vi "Q14070-Z050在线跑合.vi"() -> ()   [LabVIEW 2013]
panel:
  in  "确定按钮 3":bool
  in  "确定按钮 2":bool
  in  "密码":string
  in  "确定按钮":bool
  out "不合格":bool
  out "error out 4":errorcluster
  out "error out":errorcluster
  out "Data":string[][](array[string])
  out "型号数量":i32=10
  out "通道0":dbl
  out "I复位按钮":bool
  out "I急停按钮":bool
  out "报警信息":string
  out "电机当前位置":dbl=10000.0 format="%#.2f"
  out "拉压力（N）":dbl format="%#.1f"
  out "通讯状态":bool
  in  "停止":bool
  out "自动操作状态":string
  out "工步号":dbl
  in  "联线按钮":bool
  in  "选项卡控件 2":enum32{"自动工步", "手动气缸", "传感器校验", "参数查询"}(tab)
  out "跑和设定百分比":dbl=3.0 format="%#_2f"
  out "跑和百分比":dbl=1.0 format="%.2f"
  out "跑合已完成次数":dbl
  out "跑合速度(mm/s)":dbl=3.0 format="%#_2f"
  out "跑合设定次数":dbl=10.0
  out "左极限位置(mm)":dbl=-40.0
  out "右极限位置(mm)":dbl=60.0
  out "齿条中心位置（mm)":dbl=14.0
  out "齿条行程(mm)":dbl=14.0
  out "顶升气缸上位 2":bool
  out "顶升气缸下位 2":bool
  out "齿条夹紧 2":bool
  out "齿条松开 2":bool
  out "下工位在位  2":bool
  out "本工位在位 2":bool
  out "上工位在位  2":bool
  out "换向拉压力(N)":dbl format="%#.3f"
  out "本序合格":bool
  out "上序不合格":bool
  out "上序合格":bool
  out "本序已做":bool
  out "I齿条松开":bool
  out "I齿条夹紧":bool
  out "I顶升气缸下位":bool
  out "I顶升气缸上位":bool
  out "下工位在位":bool
  out "本工位在位":bool
  out "上工位在位":bool
  in  "M上阻挡器放行":bool
  in  "M本阻挡器放行":bool
  in  "M顶升气缸上升":bool
  in  "M顶升气缸下降":bool
  in  "M齿条气缸夹紧":bool
  in  "M齿条气缸松开":bool
  in  "电机前进":bool
  in  "电机后退":bool
  in  "电机回零":bool
  in  "拉压力1传感器零点偏移":dbl format="%#.2f"
  in  "拉压力1传感器比例偏移":dbl=1.0 format="%#.2f"
  in  "传感器参数保存":bool
  in  "参数查询":bool
  in  "参数列表":string[][](table)
  in  "参数修改":bool
  out "员工ID":string
  out "员工姓名":string
  in  "型号选择":u16(ring)=1 items=["J706", "J709", "J728"]
  in  "参数加载":bool
  out "产品ID":string
  out "报警 工步号":dbl
  out "完成":bool
  out "error out 3":errorcluster
  out "芯片ID":string
  out "error out 2":errorcluster
  out "ADODB._Connection Out":refnum<k7>
  out "跑合曲线":cluster{dbl[], dbl[]}(graph)
  out "FGCS":string
  out "RFID读取完成":bool
  out "RFID读取触发":bool
  out "05RFID":string
  out "KSJJ":string
  out "ReturnValue 3":u32
  out "ReturnValue":u32
  out "轴1AxisHandle OUT":u32
  out "DeviceHandle":u32
  # "芜湖机械转向器装配线"
  # "在线跑合"
  # "湖北唯思凌科装备制造有限公司 设计开发 (C)2015"
  # "Q14070机械转向器装配线"
  # "传感器校验区"
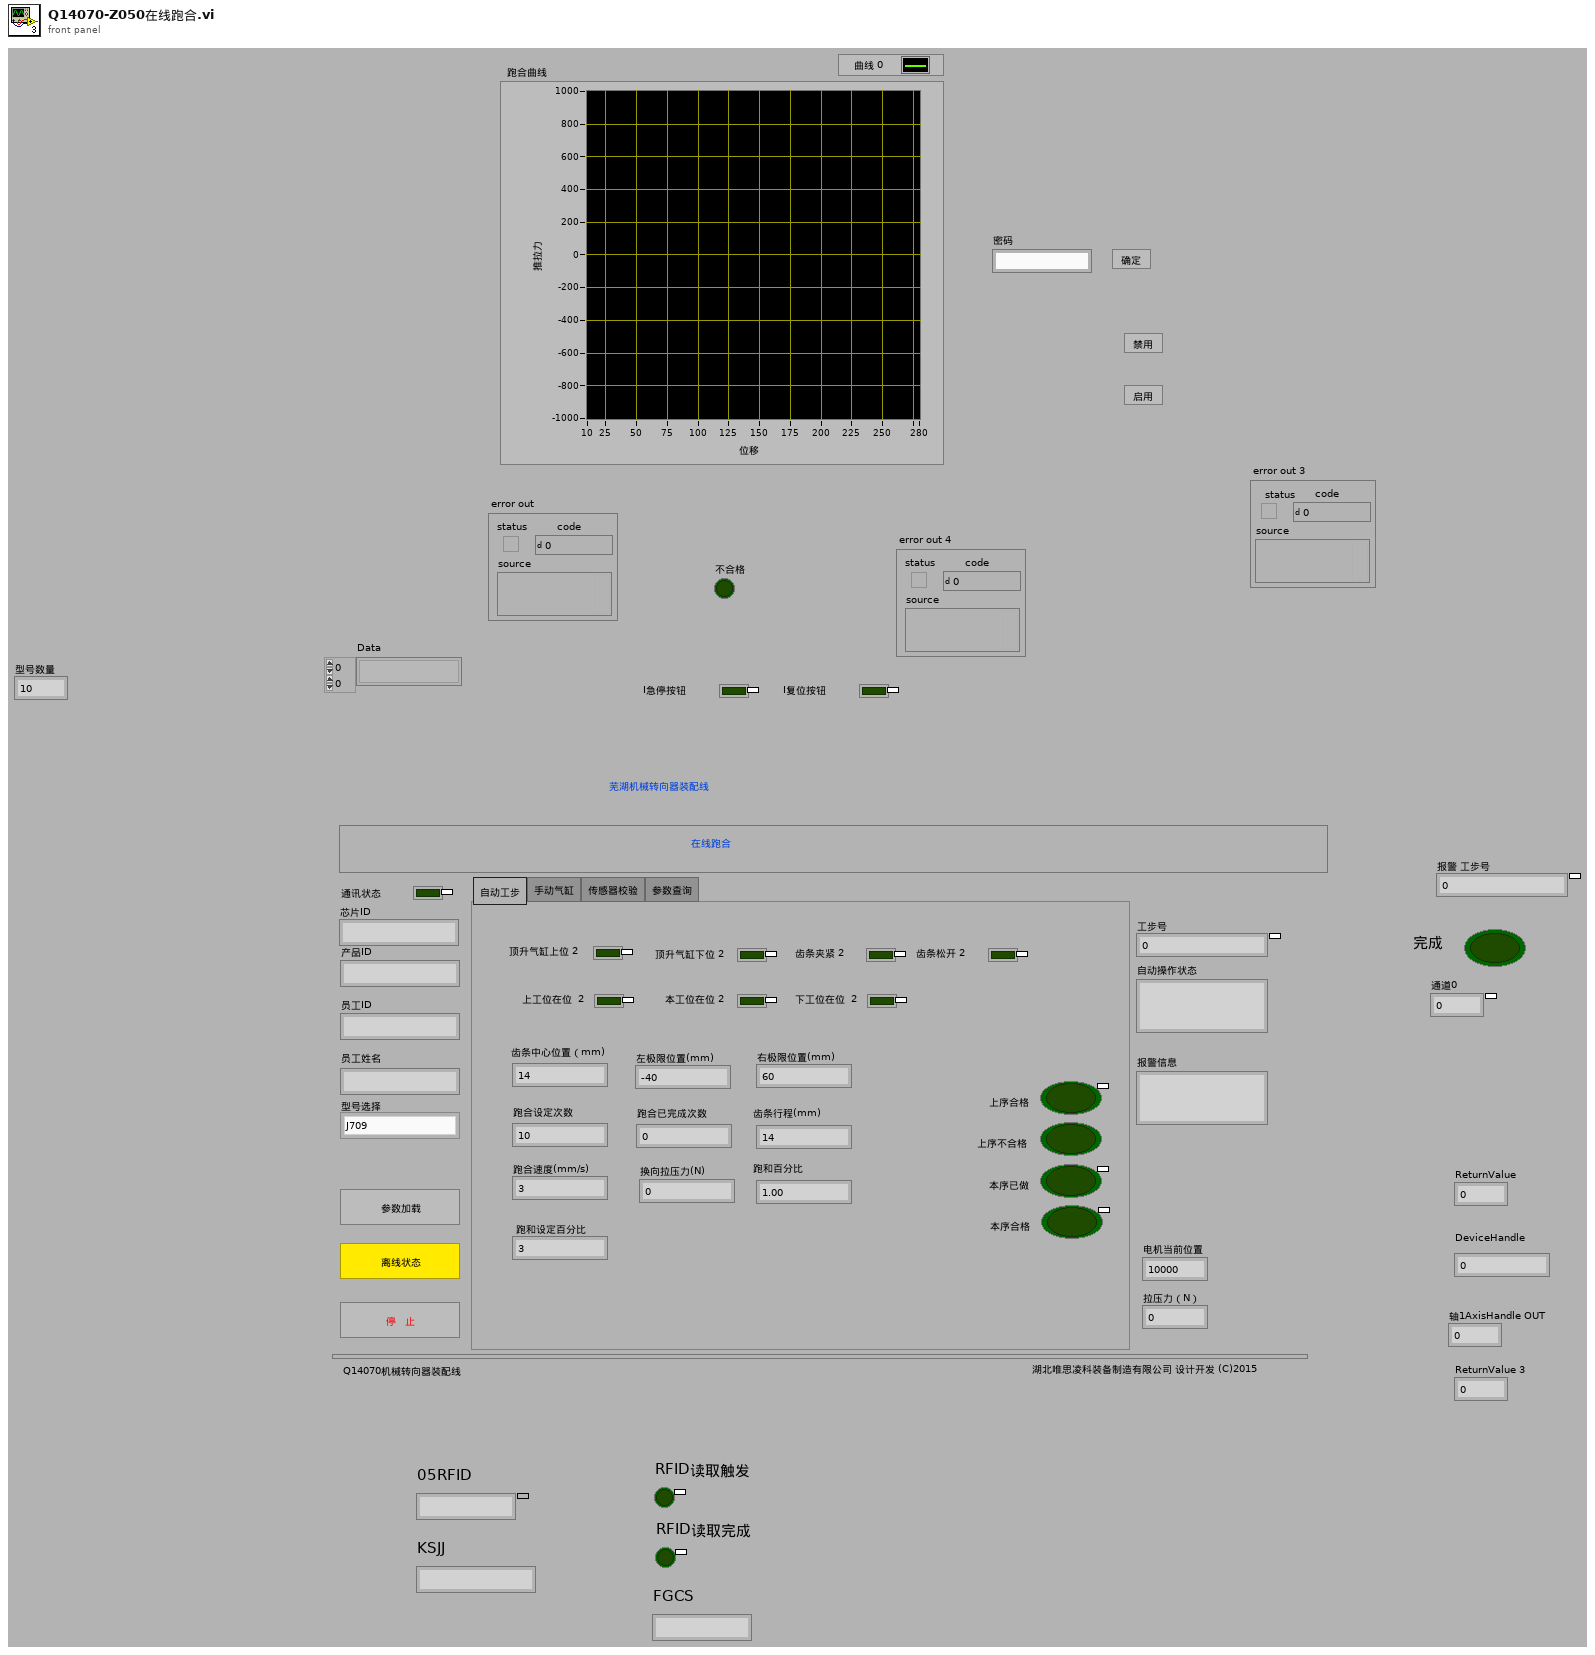
[diagram p1: front panel]
types:
  T1 = enum8{"Enabled", "Disabled", "Disabled and Grayed Out"}
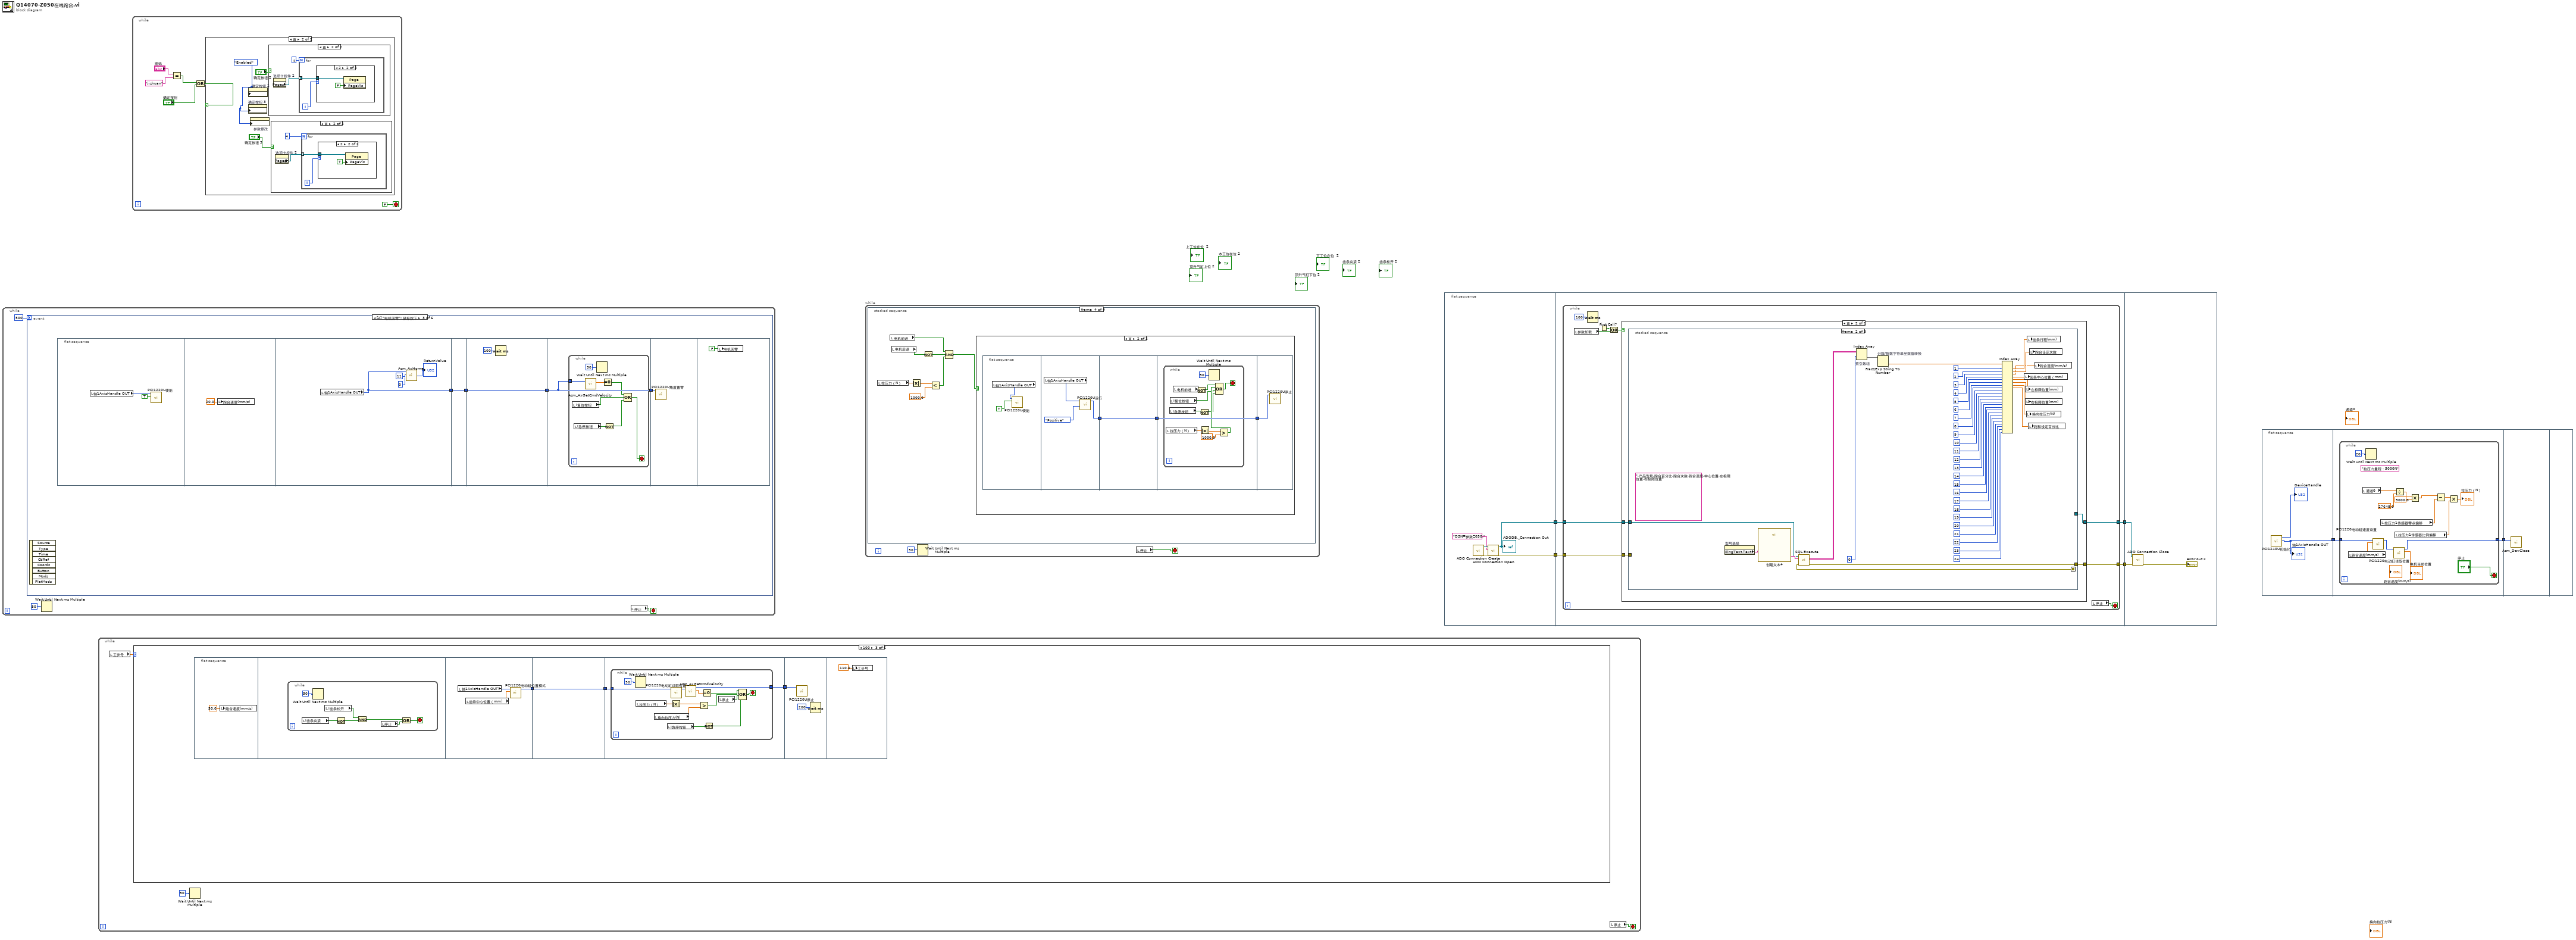
[diagram p0: block diagram]
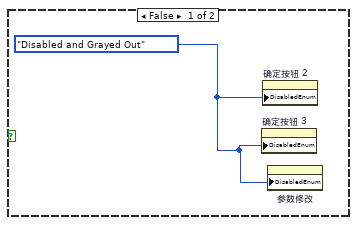
[diagram p2: hidden frame]
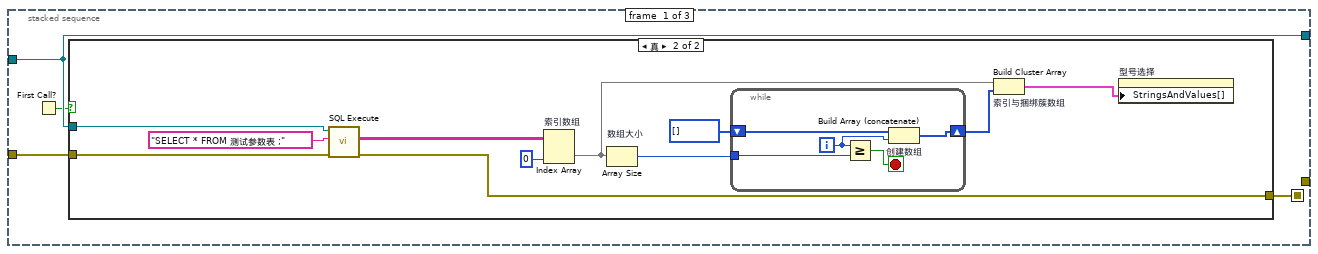
[diagram p8: hidden frame]
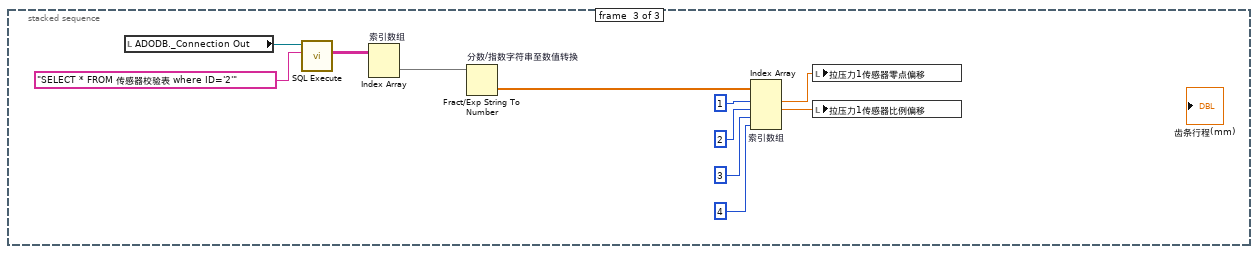
[diagram p10: hidden frame]
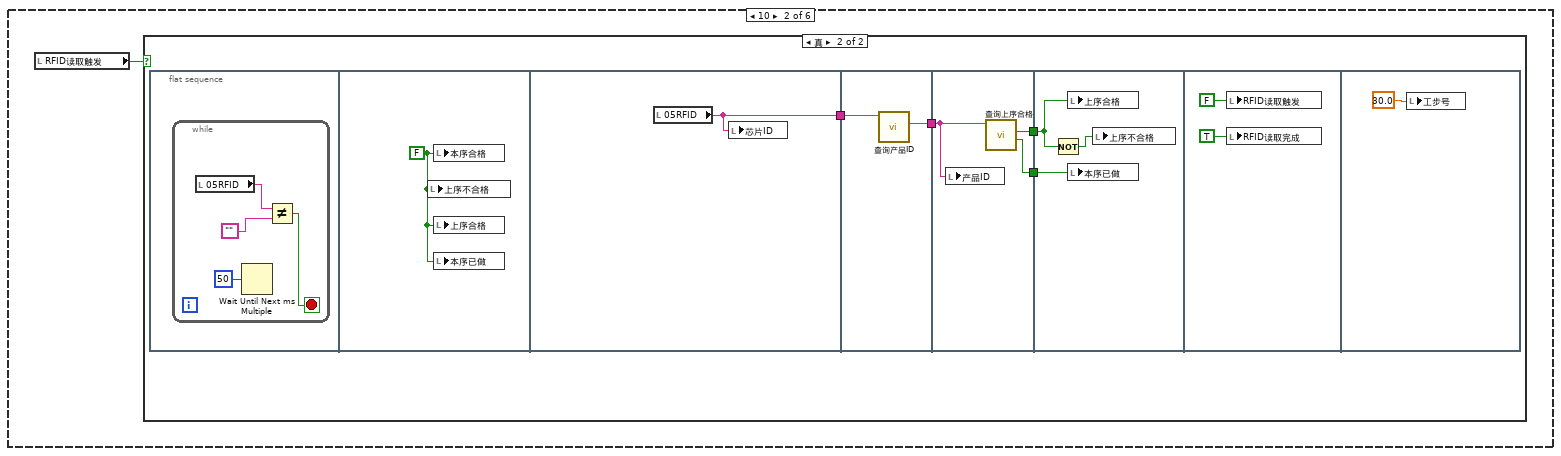
[diagram p12: hidden frame]
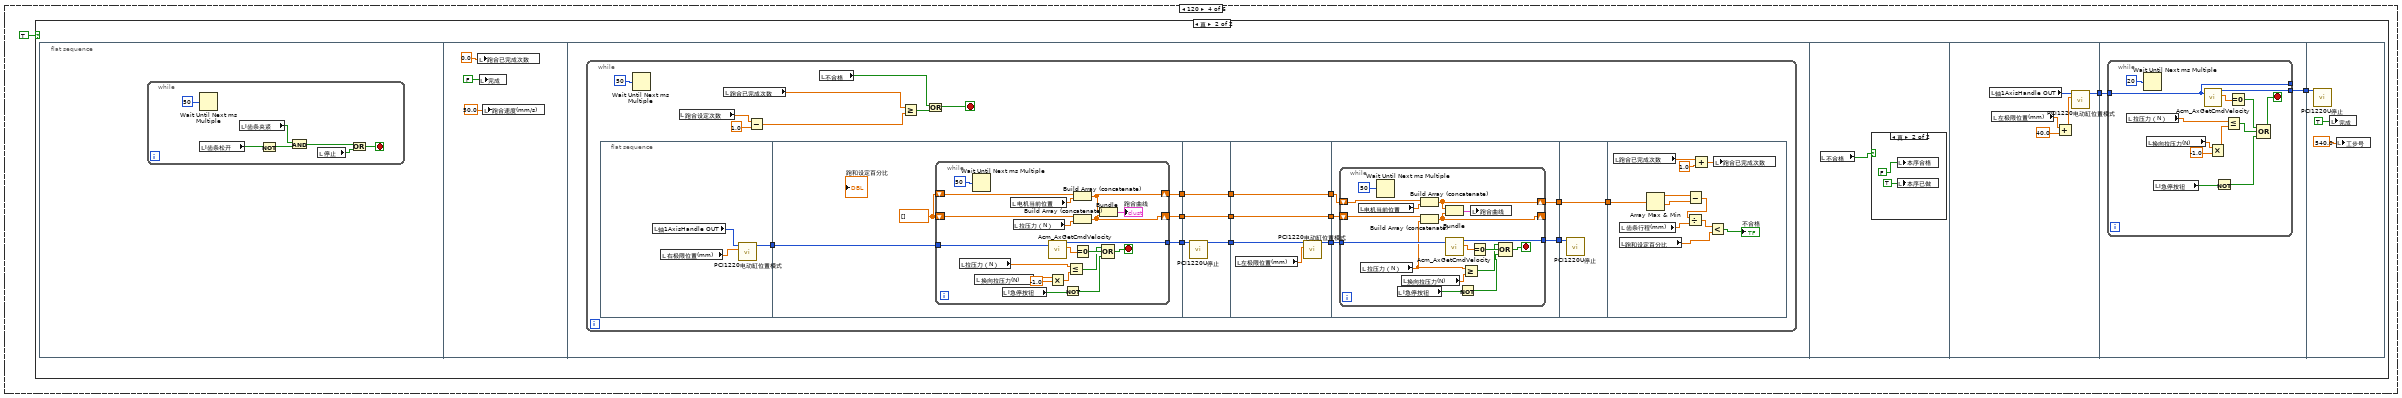
[diagram p14: hidden frame]
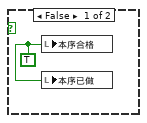
[diagram p16: hidden frame]
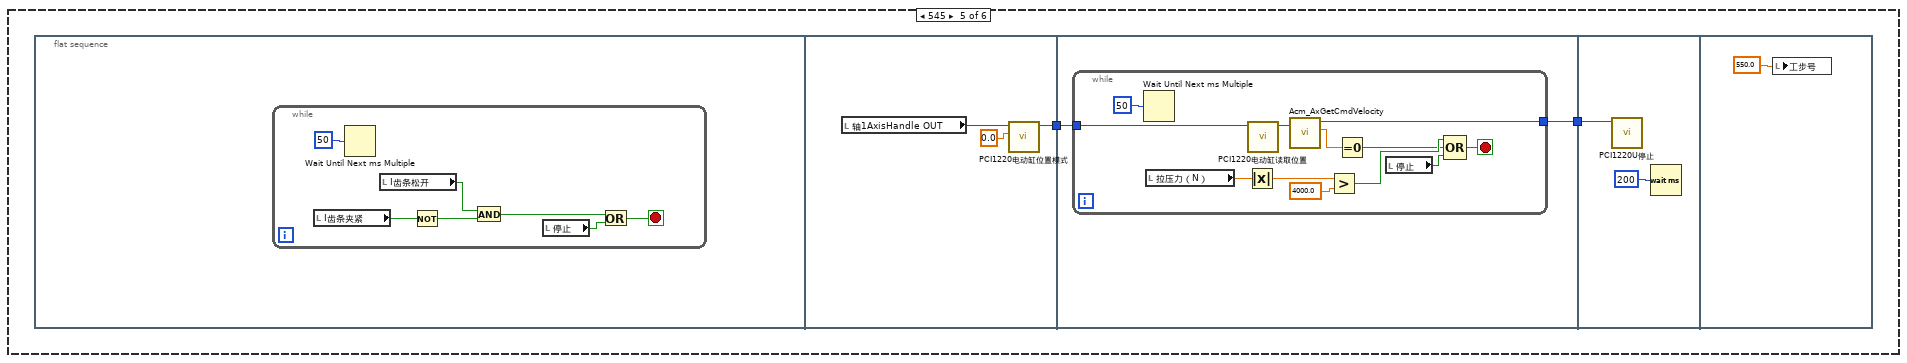
[diagram p17: hidden frame]
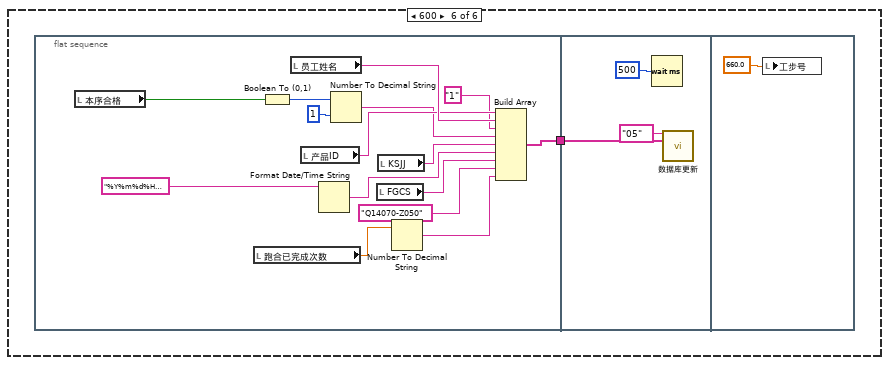
[diagram p18: hidden frame]
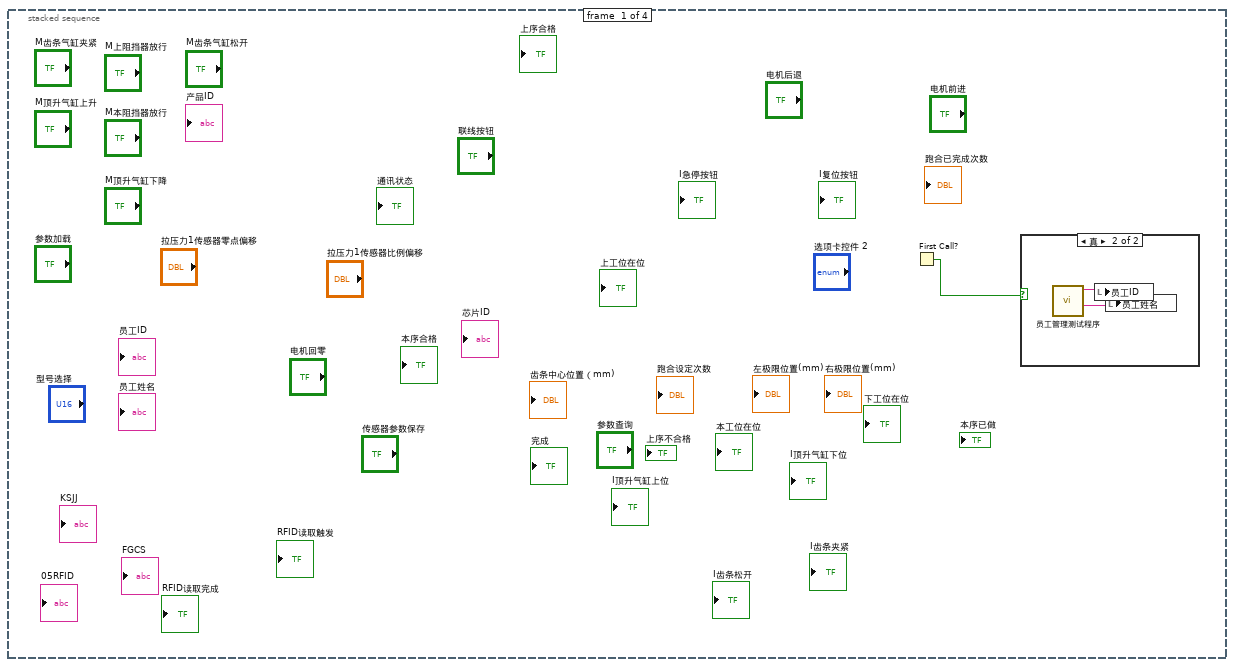
[diagram p19: hidden frame]
diagram:
  n1 = while {
    stop <- w7 stop-if-true
    n2 = event shown="[2] \"电机回零\": 鼠标按下" {
      selector: _ -> [_ _ _ _ _ _]
      dyn-events: _ -> [_ _ _ _ _ _]
      timeout: 500 -> [_ _ _ _ _ _]
      event Timeout {
        n3 = event-data() -> ()  [unwired: 3 out]
      }
      event "停止": Value Change {
        n4 = event-data() -> ()  [unwired: 7 out]
        n5 = flat-sequence {
          frame #0 {
            n6 = local write "工步号"(0.0 ("工步号")) -> ()
          }
          frame #1 {
            n7 = Wait Until Next ms Multiple(millisecond multiple=u32 1000 ("毫秒倍数")) -> ()  [unwired: 1 out]
          }
          frame #2 {
            n8 = Quit LabVIEW(quit? (T)=TRUE ("停止？(T)")) -> ()
          }
        }
      }
      event "电机回零": Mouse Down {
        n9 = event-data() -> ()  [unwired: 9 out]
        n10 = flat-sequence {
          tunnel: [w20] -> w14
          tunnel: w14 -> [w24]
          tunnel: [w24] -> w13
          tunnel: w13 -> [w25]
          tunnel: [w25] -> w15
          tunnel: w15 -> [w27]
          tunnel: [w27] -> w16
          tunnel: w16 -> [w36]
          frame #0 {
            n11 = local read "轴1AxisHandle OUT"() -> (w18:u32)
            n12 = call "PCI1220U使能.vi"("使能"=TRUE, "AxisHandle IN"=w18) -> ()  [unwired: 9 in, 1 out]
          }
          frame #1 {
            n13 = local write "跑合速度(mm/s)"(20.0 ("跑合速度(mm/s)")) -> ()
          }
          frame #2 {
            n14 = local read "轴1AxisHandle OUT"() -> (w20:u32)
            n15 = call <userlib>:"Acm_AxHome.vi"("DirMode"=u32 0, "HomeMode"=u32 11, "AxisHandle"=w20) -> ("ReturnValue"=→"ReturnValue":u32)  [unwired: 1 in, 2 out]
          }
          frame #3 {
          }
          frame #4 {
            n16 = Wait (ms)(milliseconds to wait=u32 100 ("毫秒倍数")) -> ()  [unwired: 1 out]
          }
          frame #5 {
            n17 = while {
              tunnel: w27 -> [w35]
              stop <- w28 stop-if-true
              n18 = local read "I复位按钮"() -> (w30:bool)
              n19 = local read "I急停按钮"() -> (w32:bool)
              n20 = call <userlib>:"Acm_AxGetCmdVelocity.vi"("AxisHandle"=w35) -> ("Velocity"=w34:dbl)  [unwired: 1 in, 3 out]
              n21 = Wait Until Next ms Multiple(millisecond multiple=u32 50 ("毫秒倍数")) -> ()  [unwired: 1 out]
              n22 = Equal To 0?(x=w34) -> (x = 0?=w31:bool)
              n23 = Not(x=w32) -> (.not. x?=w29:bool)
              n24 = Compound Arithmetic op=OR(w31, w30, w29) -> (w28:bool)
            }
          }
          frame #6 {
            n25 = call "PCI1220U角度置零.vi"("AxisHandle IN"=w36) -> ()  [unwired: 10 in, 1 out]
          }
          frame #7 {
            n26 = local write "电机回零"(FALSE ("回零")) -> ()
          }
        }
      }
      event "参数查询": Value Change {
        n27 = event-data() -> ()  [unwired: 7 out]
        n28 = flat-sequence {
          tunnel: [w46] -> w43
          tunnel: [w56] -> w42
          tunnel: [w52] -> w41
          tunnel: [w49] -> w40
          tunnel: w43 -> [w61]
          tunnel: w42 -> [w59]
          tunnel: [w60] -> w39
          tunnel: w41 -> [w60]
          tunnel: [w59] -> w38
          tunnel: w40 -> [w58]
          tunnel: w39 -> [w64]
          tunnel: w38 -> [w63]
          frame #0 {
            n29 = call "字符串转换为数组.vi"("查询内容"=",产品型号,齿条行程,跑合次数,跑合速度,中心位置,左极限位置,右极限位置,换向拉压力,跑和设定百分比") -> ("列首"=w44:string[])  [unwired: 10 in]
            n30 = property on="参数列表" class="Tbl (严格)"("Row Headers[]"=w44) -> ()  [unwired: 2 in, 2 out]
          }
          frame #1 {
            n31 = call "创建文本"() -> ("Result"=w57:string)  [unwired: 14 in, 1 out]
            n32 = call "ADO Connection Create.vi"() -> ("error out"=w51:errorcluster, "ADODB._Connection Out"=w55:refnum<k7>)  [unwired: 10 in]
            n33 = call "ADO Connection Open.vi"("error in (no error)"=w51, "ConnectionString"="DSN=参数Z050;", "ADODB._Connection In"=w55) -> ("error out"=w50:errorcluster, "ADODB._Connection Out"=w53:refnum<k7>)  [unwired: 7 in]
            n34 = call "SQL Execute.vi"("error in (no error)"=w50, "Command Text"=w57, "ADODB._Connection In"=w53) -> ("error out"=w56:errorcluster, "Data"=w48:string[][], "ADODB._Connection Out"=w52:refnum<k7>)  [unwired: 5 in, 1 out]
            n35 = Transpose 2D Array "二维数组转置"(2D array=w48) -> (transposed array=w46:string[][])
            n36 = Index Array(array=w46, index (row)=0 ("索引 (行)")) -> (element=w49:string[])  [unwired: 1 in]
          }
          frame #2 {
            n37 = local write "参数列表"(w61) -> ()
            n38 = property on="参数列表" class="Tbl (严格)"("Column Headers[]"=w58) -> ()  [unwired: 2 in, 2 out]
          }
          frame #3 {
            n39 = call "ADO Connection Close.vi"("error in (no error)"=w63, "ADODB._Connection In"=w64) -> ("error out"=→"error out 4":errorcluster)  [unwired: 8 in, 1 out]
          }
        }
      }
      event "传感器参数保存": Value Change {
        n40 = event-data() -> ()  [unwired: 7 out]
        n41 = local read "拉压力1传感器零点偏移"() -> (w65:dbl)
        n42 = local read "拉压力1传感器比例偏移"() -> (w66:dbl)
        n43 = call "ADO Connection Create.vi"() -> ("error out"=w75:errorcluster, "ADODB._Connection Out"=w77:refnum<k7>)  [unwired: 10 in]
        n44 = Number To Fractional String(number=w65, precision (6)=i16 3 ("精度(6)")) -> (F-format string=w70:string)  [unwired: 2 in]
        n45 = Number To Fractional String(number=w66, precision (6)=i16 2 ("精度(6)")) -> (F-format string=w69:string)  [unwired: 2 in]
        n46 = call "创建文本3"("拉压力1传感器零点偏移"=w70, "拉压力1传感器比例偏移"=w69) -> ("Result"=w68:string)  [unwired: 12 in, 1 out]
        n47 = call "ADO Connection Open.vi"("error in (no error)"=w75, "ConnectionString"="DSN=参数Z050;", "ADODB._Connection In"=w77) -> ("error out"=w74:errorcluster, "ADODB._Connection Out"=w76:refnum<k7>)  [unwired: 7 in]
        n48 = call "SQL Execute.vi"("error in (no error)"=w74, "Command Text"=w68, "ADODB._Connection In"=w76) -> ("error out"=w78:errorcluster, "ADODB._Connection Out"=w79:refnum<k7>)  [unwired: 5 in, 2 out]
        n49 = call "ADO Connection Close.vi"("error in (no error)"=w78, "ADODB._Connection In"=w79) -> ("error out"=→"error out 3":errorcluster)  [unwired: 8 in, 1 out]
      }
      event "参数修改": Value Change {
        n50 = event-data() -> ()  [unwired: 7 out]
        n51 = while {
          i -> [w111]
          stop <- w110 stop-if-true
          (unwired) "UPDATE 测试参数表 SET 齿条行程='%齿条行程%',跑合次数='%跑合次数%',跑合速度='%跑合速度%',中心位置='%中心位置%' ,左极限位置='%左极限位置%' ,右极限位置='%右极限位置%' ,换向拉压力='%换向拉压力%' WHERE 产品型号 = '%产品型号%';"
          (unwired) 11 ("索引")
          (unwired) 10 ("索引")
          n52 = local read "参数列表"() -> (w113:string[][])
          n53 = local read "型号数量"() -> (w112:i32)
          n54 = Wait Until Next ms Multiple(millisecond multiple=u32 100 ("毫秒倍数")) -> ()  [unwired: 1 out]
          n55 = Greater Or Equal?(x=w111, y=w112) -> (x >= y?=w110:bool)
          n56 = Index Array(array=w113, index (col)=w111) -> (element=w105:string[])  [unwired: 1 in]
          n57 = Index Array(array=w105, index #1=1 ("索引"), index #2=2 ("索引"), index #3=3 ("索引"), index #4=4 ("索引"), index #5=5 ("索引"), index #6=6 ("索引"), index #7=7 ("索引"), index #8=8 ("索引"), index #9=0 ("索引")) -> (element #1=w88:string, element #2=w87:string, element #3=w86:string, element #4=w85:string, element #5=w84:string, element #6=w83:string, element #7=w82:string, element #8=w81:string, element #9=w80:string)
          n58 = call "创建文本2"("齿条行程"=w88, "跑合次数"=w87, "跑合速度"=w86, "中心位置"=w85, "左极限位置"=w84, "右极限位置"=w83, "换向拉压力"=w82, "跑和设定百分比"=w81, "产品型号"=w80) -> ("Result"=w89:string)  [unwired: 17 in, 1 out]
          n59 = call "ADO Connection Create.vi"("error in (no error)"=errorcluster {"status"=FALSE, "code"=0, "source"=""}) -> ("error out"=w97:errorcluster, "ADODB._Connection Out"=w99:refnum<k7>)  [unwired: 9 in]
          n60 = call "ADO Connection Open.vi"("error in (no error)"=w97, "ConnectionString"="DSN=参数Z050;", "ADODB._Connection In"=w99) -> ("error out"=w96:errorcluster, "ADODB._Connection Out"=w98:refnum<k7>)  [unwired: 7 in]
          n61 = call "SQL Execute.vi"("error in (no error)"=w96, "Command Text"=w89, "ADODB._Connection In"=w98) -> ("error out"=w103:errorcluster, "Data"=→"Data":string[][], "ADODB._Connection Out"=w104:refnum<k7>)  [unwired: 5 in, 1 out]
          n62 = call "ADO Connection Close.vi"("error in (no error)"=w103, "ADODB._Connection In"=w104) -> ("error out"=→"error out":errorcluster)  [unwired: 8 in, 1 out]
        }
      }
    }
    n63 = Wait Until Next ms Multiple(millisecond multiple=u32 50 ("毫秒倍数")) -> ()  [unwired: 1 out]
    n64 = local read "停止"() -> (w7:bool)
  }
  n65 = while {
    stop <- w117 stop-if-true
    n66 = local read "工步号"() -> (w115:dbl)
    n67 = case shown="100" w115 {
      frame 0, Default {
      }
      frame 10 {
        n68 = local read "RFID读取触发"() -> (w118:bool)
        n69 = case shown="真" w118 {
          frame False {
          }
          frame True {
            n70 = flat-sequence {
              tunnel: [w128] -> w122
              tunnel: w122 -> [w130]
              tunnel: [w129] -> w121
              tunnel: w121 -> [w133]
              tunnel: [w132] -> w120
              tunnel: [w131] -> w119
              tunnel: w120 -> [w135]
              tunnel: w119 -> [w136]
              frame #0 {
                n71 = while {
                  stop <- w124 stop-if-true
                  n72 = local read "05RFID"() -> (w126:string)
                  n73 = Wait Until Next ms Multiple(millisecond multiple=u32 50 ("毫秒倍数")) -> ()  [unwired: 1 out]
                  n74 = Not Equal?(x=w126, y="") -> (x != y?=w124:bool)
                }
              }
              frame #1 {
                w127 = FALSE ("本序合格")
                n75 = local write "上序不合格"(w127) -> ()
                n76 = local write "本序合格"(w127) -> ()
                n77 = local write "上序合格"(w127) -> ()
                n78 = local write "本序已做"(w127) -> ()
              }
              frame #2 {
                n79 = local read "05RFID"() -> (w128:string)
                n80 = local write "芯片ID"(w128) -> ()
              }
              frame #3 {
                n81 = call "查询产品ID.vi"("芯片编码"=w130) -> ("产品ID"=w129:string)  [unwired: 8 in, 2 out]
              }
              frame #4 {
                n82 = local write "产品ID"(w133) -> ()
                n83 = call "查询上序合格.vi"("产品ID"=w133) -> ("本序已做"=w131:bool, "上序合格"=w132:bool)  [unwired: 8 in, 1 out]
              }
              frame #5 {
                n84 = Not(x=w135) -> (.not. x?=w134:bool)
                n85 = local write "上序合格"(w135) -> ()
                n86 = local write "本序已做"(w136) -> ()
                n87 = local write "上序不合格"(w134) -> ()
              }
              frame #6 {
                n88 = local write "RFID读取触发"(FALSE ("RFID读取触发")) -> ()
                n89 = local write "RFID读取完成"(TRUE ("RFID读取完成")) -> ()
              }
              frame #7 {
                n90 = local write "工步号"(30.0 ("工步号")) -> ()
              }
            }
          }
        }
      }
      frame 100 {
        n91 = flat-sequence {
          tunnel: [w151] -> w141
          tunnel: w141 -> [w154]
          tunnel: [w154] -> w140
          tunnel: w140 -> [w156]
          tunnel: [w155] -> w142
          tunnel: w142 -> [w172]
          frame #0 {
            n92 = local write "跑合速度(mm/s)"(50.0 ("跑合速度(mm/s)")) -> ()
          }
          frame #1 {
            n93 = while {
              stop <- w144 stop-if-true
              n94 = local read "I齿条夹紧"() -> (w149:bool)
              n95 = Wait Until Next ms Multiple(millisecond multiple=u32 50 ("毫秒倍数")) -> ()  [unwired: 1 out]
              n96 = local read "I齿条松开"() -> (w148:bool)
              n97 = Not(x=w149) -> (.not. x?=w147:bool)
              n98 = And(x=w148, y=w147) -> (x .and. y?=w146:bool)
              n99 = local read "停止"() -> (w145:bool)
              n100 = Or(x=w146, y=w145) -> (x .or. y?=w144:bool)
            }
          }
          frame #2 {
            n101 = local read "轴1AxisHandle OUT"() -> (w152:u32)
            n102 = local read "齿条中心位置（mm)"() -> (w153:dbl)
            n103 = call "PCI1220电动缸位置模式 .vi"("Distance"=w153, "AxisHandle IN"=w152) -> ("AxisHandle OUT"=w151:u32)  [unwired: 8 in, 1 out]
          }
          frame #3 {
          }
          frame #4 {
            n104 = while {
              tunnel: [w166] -> w155
              tunnel: w156 -> [w165]
              stop <- w161 stop-if-true
              n105 = Wait Until Next ms Multiple(millisecond multiple=u32 50 ("毫秒倍数")) -> ()  [unwired: 1 out]
              n106 = local read "拉压力（N）"() -> (w168:dbl)
              n107 = local read "换向拉压力(N)"() -> (w157:dbl)
              n108 = local read "I急停按钮"() -> (w159:bool)
              n109 = Absolute Value(x=w168) -> (abs(x)=w167:dbl)
              n110 = call "PCI1220电动缸读取位置.vi"("AxisHandle IN"=w165) -> ("AxisHandle OUT"=w164:u32)  [unwired: 9 in, 1 out]
              n111 = call <userlib>:"Acm_AxGetCmdVelocity.vi"("AxisHandle"=w164) -> ("Velocity"=w170:dbl, "AxisHandle"=w166:u32)  [unwired: 1 in, 2 out]
              n112 = Greater?(x=w167, y=w157) -> (0:w163:bool)
              n113 = Equal To 0?(x=w170) -> (x = 0?=w162:bool)
              n114 = Not(x=w159) -> (.not. x?=w158:bool)
              n115 = local read "停止"() -> (w160:bool)
              n116 = Compound Arithmetic op=OR(w163, w162, w160, w158) -> (w161:bool)
            }
          }
          frame #5 {
            n117 = call "PCI1220U停止.vi"("AxisHandle IN"=w172) -> ()  [unwired: 9 in, 2 out]
            n118 = Wait (ms)(milliseconds to wait=u32 200 ("等待时间（毫秒）")) -> ()  [unwired: 1 out]
          }
          frame #6 {
            n119 = local write "工步号"(110.0 ("工步号")) -> ()
          }
        }
      }
      frame 120 {
        n120 = case shown="真" TRUE {
          frame False {
          }
          frame True {
            n121 = flat-sequence {
              tunnel: [w287] -> w176
              tunnel: w176 -> [w290]
              tunnel: [w289] -> w175
              tunnel: w175 -> [w306]
              frame #0 {
                n122 = while {
                  stop <- w177 stop-if-true
                  n123 = Wait Until Next ms Multiple(millisecond multiple=u32 50 ("毫秒倍数")) -> ()  [unwired: 1 out]
                  n124 = local read "I齿条松开"() -> (w182:bool)
                  n125 = local read "I齿条夹紧"() -> (w181:bool)
                  n126 = Not(x=w182) -> (.not. x?=w180:bool)
                  n127 = And(x=w181, y=w180) -> (x .and. y?=w179:bool)
                  n128 = local read "停止"() -> (w178:bool)
                  n129 = Or(x=w179, y=w178) -> (x .or. y?=w177:bool)
                }
              }
              frame #1 {
                n130 = local write "跑合已完成次数"(0.0 ("已完成次数")) -> ()
                n131 = local write "完成"(FALSE ("完成")) -> ()
                n132 = local write "跑合速度(mm/s)"(50.0 ("跑合速度(mm/s)")) -> ()
              }
              frame #2 {
                n133 = while {
                  stop <- w188 stop-if-true
                  n134 = flat-sequence {
                    tunnel: [w209] -> w206
                    tunnel: w206 -> [w215]
                    tunnel: [w214] -> w205
                    tunnel: [w212] -> w197
                    tunnel: [w211] -> w194
                    tunnel: w205 -> [w239]
                    tunnel: [w238] -> w204
                    tunnel: [w237] -> w198
                    tunnel: w197 -> [w237]
                    tunnel: [w236] -> w195
                    tunnel: w194 -> [w236]
                    tunnel: w204 -> [w244]
                    tunnel: [w243] -> w203
                    tunnel: [w242] -> w199
                    tunnel: w198 -> [w242]
                    tunnel: [w241] -> w196
                    tunnel: w195 -> [w241]
                    tunnel: w203 -> [w249]
                    tunnel: [w248] -> w202
                    tunnel: w199 -> [w247]
                    tunnel: w196 -> [w246]
                    tunnel: [w245] -> w189
                    tunnel: w202 -> [w268]
                    tunnel: [w267] -> w190
                    tunnel: w189 -> [w267]
                    tunnel: w190 -> [w276]
                    frame #0 {
                      n135 = local read "轴1AxisHandle OUT"() -> (w210:u32)
                      n136 = local read "右极限位置(mm)"() -> (w208:dbl)
                      n137 = call "PCI1220电动缸位置模式 .vi"("Distance"=w208, "AxisHandle IN"=w210) -> ("AxisHandle OUT"=w209:u32)  [unwired: 8 in, 1 out]
                    }
                    frame #1 {
                      w213 = dbl[] [] ("添加的数组")
                      n138 = while {
                        tunnel: w215 -> [w223]
                        tunnel: [w233] -> w214
                        shift-right: [w228] -> w212
                        shift-left: w213 -> [w231]
                        shift-right: [w227] -> w211
                        shift-left: w213 -> [w229]
                        stop <- w224 stop-if-true
                        n139 = local read "拉压力（N）"() -> (w217:dbl)
                        n140 = Wait Until Next ms Multiple(millisecond multiple=u32 50 ("毫秒倍数")) -> ()  [unwired: 1 out]
                        n141 = local read "换向拉压力(N)"() -> (w220:dbl)
                        n142 = local read "I急停按钮"() -> (w222:bool)
                        n143 = local read "电机当前位置"() -> (w232:dbl)
                        n144 = local read "拉压力（N）"() -> (w230:dbl)
                        n145 = call <userlib>:"Acm_AxGetCmdVelocity.vi"("AxisHandle"=w223) -> ("Velocity"=w235:dbl, "AxisHandle"=w233:u32)  [unwired: 1 in, 2 out]
                        n146 = Multiply(x=w220, y=-1.0) -> (x*y=w218:dbl)
                        n147 = Not(x=w222) -> (.not. x?=w221:bool)
                        n148 = Less Or Equal?(x=w217, y=w218) -> (x <= y?=w216:bool)
                        n149 = Build Array (concatenate)(w231, w232) -> (w228:dbl[])
                        n150 = Build Array (concatenate)(w229, w230) -> (w227:dbl[])
                        n151 = Equal To 0?(x=w235) -> (x = 0?=w225:bool)
                        n152 = Bundle(w228, w227) -> (→"跑合曲线":cluster{dbl[], dbl[]})  [unwired: 1 in]
                        n153 = Compound Arithmetic op=OR(w216, w225, w221) -> (w224:bool)
                      }
                    }
                    frame #2 {
                      n154 = call "PCI1220U停止.vi"("AxisHandle IN"=w239) -> ("AxisHandle OUT"=w238:u32)  [unwired: 9 in, 1 out]
                    }
                    frame #3 {
                      n155 = local read "左极限位置(mm)"() -> (w240:dbl)
                      n156 = call "PCI1220电动缸位置模式 .vi"("Distance"=w240, "AxisHandle IN"=w244) -> ("AxisHandle OUT"=w243:u32)  [unwired: 8 in, 1 out]
                    }
                    frame #4 {
                      n157 = while {
                        tunnel: w249 -> [w266]
                        tunnel: [w263] -> w248
                        shift-right: [w259] -> w245
                        shift-left: w247 -> [w262]
                        shift-right: [w258] -> _
                        shift-left: w246 -> [w261]
                        stop <- w255 stop-if-true
                        n158 = local read "电机当前位置"() -> (w260:dbl)
                        n159 = local read "拉压力（N）"() -> (w252:dbl)
                        n160 = Wait Until Next ms Multiple(millisecond multiple=u32 50 ("毫秒倍数")) -> ()  [unwired: 1 out]
                        n161 = local read "I急停按钮"() -> (w254:bool)
                        n162 = local read "换向拉压力(N)"() -> (w251:dbl)
                        n163 = Build Array (concatenate)(w262, w260) -> (w259:dbl[])
                        n164 = Build Array (concatenate)(w261, w252) -> (w258:dbl[])
                        n165 = Bundle(w259, w258) -> (w257:cluster{dbl[], dbl[]})  [unwired: 1 in]
                        n166 = call <userlib>:"Acm_AxGetCmdVelocity.vi"("AxisHandle"=w266) -> ("Velocity"=w265:dbl, "AxisHandle"=w263:u32)  [unwired: 1 in, 2 out]
                        n167 = Not(x=w254) -> (.not. x?=w253:bool)
                        n168 = Greater Or Equal?(x=w252, y=w251) -> (x >= y?=w250:bool)
                        n169 = local write "跑合曲线"(w257) -> ()
                        n170 = Equal To 0?(x=w265) -> (x = 0?=w256:bool)
                        n171 = Compound Arithmetic op=OR(w250, w256, w253) -> (w255:bool)
                      }
                    }
                    frame #5 {
                      n172 = call "PCI1220U停止.vi"("AxisHandle IN"=w268) -> ()  [unwired: 9 in, 2 out]
                    }
                    frame #6 {
                      n173 = local read "跑合已完成次数"() -> (w279:dbl)
                      n174 = local read "跑和设定百分比"() -> (w269:dbl)
                      n175 = local read "齿条行程(mm)"() -> (w272:dbl)
                      n176 = Array Max & Min(array=w276) -> (max value=w275:dbl, min value=w274:dbl)  [unwired: 2 out]
                      n177 = Subtract(x=w275, y=w274) -> (x-y=w273:dbl)
                      n178 = Divide(x=w273, y=w272) -> (x/y=w271:dbl)
                      n179 = Add(x=w279, y=1.0) -> (x+y=w277:dbl)
                      n180 = Less?(x=w271, y=w269) -> (x < y?=→"不合格":bool)
                      n181 = local write "跑合已完成次数"(w277) -> ()
                    }
                  }
                  n182 = Wait Until Next ms Multiple(millisecond multiple=u32 50 ("等待时间（毫秒）")) -> ()  [unwired: 1 out]
                  n183 = local read "跑合设定次数"() -> (w193:dbl)
                  n184 = local read "跑合已完成次数"() -> (w201:dbl)
                  n185 = Subtract(x=w193, y=1.0) -> (x-y=w191:dbl)
                  n186 = local read "不合格"() -> (w187:bool)
                  n187 = Greater Or Equal?(x=w201, y=w191) -> (x >= y?=w200:bool)
                  n188 = Or(x=w187, y=w200) -> (x .or. y?=w188:bool)
                }
              }
              frame #3 {
                n189 = local read "不合格"() -> (w280:bool)
                n190 = case shown="真" w280 {
                  frame False {
                    w281 = TRUE
                    n191 = local write "本序合格"(w281) -> ()
                    n192 = local write "本序已做"(w281) -> ()
                  }
                  frame True {
                    n193 = local write "本序合格"(FALSE) -> ()
                    n194 = local write "本序已做"(TRUE ("本序已做")) -> ()
                  }
                }
              }
              frame #4 {
                n195 = local read "轴1AxisHandle OUT"() -> (w288:u32)
                n196 = local read "左极限位置(mm)"() -> (w286:dbl)
                n197 = Add(x=w286, y=40.0) -> (x+y=w284:dbl)
                n198 = call "PCI1220电动缸位置模式 .vi"("Distance"=w284, "AxisHandle IN"=w288) -> ("AxisHandle OUT"=w287:u32)  [unwired: 8 in, 1 out]
              }
              frame #5 {
                n199 = while {
                  tunnel: [w300] -> _
                  tunnel: [w301] -> w289
                  tunnel: w290 -> [w300]
                  stop <- w296 stop-if-true
                  n200 = local read "拉压力（N）"() -> (w295:dbl)
                  n201 = Wait Until Next ms Multiple(millisecond multiple=u32 20 ("毫秒倍数")) -> ()  [unwired: 1 out]
                  n202 = local read "换向拉压力(N)"() -> (w294:dbl)
                  n203 = local read "I急停按钮"() -> (w299:bool)
                  n204 = call <userlib>:"Acm_AxGetCmdVelocity.vi"("AxisHandle"=w300) -> ("Velocity"=w303:dbl, "AxisHandle"=w301:u32)  [unwired: 1 in, 2 out]
                  n205 = Multiply(x=w294, y=-1.0) -> (x*y=w292:dbl)
                  n206 = Not(x=w299) -> (.not. x?=w297:bool)
                  n207 = Less Or Equal?(x=w295, y=w292) -> (x <= y?=w291:bool)
                  n208 = Equal To 0?(x=w303) -> (x = 0?=w298:bool)
                  n209 = Compound Arithmetic op=OR(w298, w291, w297) -> (w296:bool)
                }
              }
              frame #6 {
                n210 = call "PCI1220U停止.vi"("AxisHandle IN"=w306) -> ()  [unwired: 9 in, 2 out]
                n211 = local write "完成"(TRUE ("完成")) -> ()
                n212 = local write "工步号"(540.0 ("工步号")) -> ()
              }
            }
          }
        }
      }
      frame 545 {
        n213 = flat-sequence {
          tunnel: [w317] -> w308
          tunnel: w308 -> [w320]
          tunnel: [w319] -> w307
          tunnel: w307 -> [w334]
          frame #0 {
            n214 = while {
              stop <- w309 stop-if-true
              n215 = local read "I齿条夹紧"() -> (w314:bool)
              n216 = Wait Until Next ms Multiple(millisecond multiple=u32 50 ("毫秒倍数")) -> ()  [unwired: 1 out]
              n217 = local read "I齿条松开"() -> (w313:bool)
              n218 = Not(x=w314) -> (.not. x?=w312:bool)
              n219 = And(x=w313, y=w312) -> (x .and. y?=w311:bool)
              n220 = local read "停止"() -> (w310:bool)
              n221 = Or(x=w311, y=w310) -> (x .or. y?=w309:bool)
            }
          }
          frame #1 {
            n222 = local read "轴1AxisHandle OUT"() -> (w318:u32)
            n223 = call "PCI1220电动缸位置模式 .vi"("Distance"=0.0, "AxisHandle IN"=w318) -> ("AxisHandle OUT"=w317:u32)  [unwired: 8 in, 1 out]
          }
          frame #2 {
            n224 = while {
              tunnel: [w327] -> w319
              tunnel: w320 -> [w326]
              stop <- w322 stop-if-true
              n225 = Wait Until Next ms Multiple(millisecond multiple=u32 50 ("毫秒倍数")) -> ()  [unwired: 1 out]
              n226 = local read "拉压力（N）"() -> (w330:dbl)
              n227 = Absolute Value(x=w330) -> (abs(x)=w329:dbl)
              n228 = call "PCI1220电动缸读取位置.vi"("AxisHandle IN"=w326) -> ("AxisHandle OUT"=w325:u32)  [unwired: 9 in, 1 out]
              n229 = call <userlib>:"Acm_AxGetCmdVelocity.vi"("AxisHandle"=w325) -> ("Velocity"=w332:dbl, "AxisHandle"=w327:u32)  [unwired: 1 in, 2 out]
              n230 = Greater?(x=w329, y=4000.0) -> (0:w324:bool)
              n231 = Equal To 0?(x=w332) -> (x = 0?=w323:bool)
              n232 = local read "停止"() -> (w321:bool)
              n233 = Compound Arithmetic op=OR(w324, w323, w321) -> (w322:bool)
            }
          }
          frame #3 {
            n234 = call "PCI1220U停止.vi"("AxisHandle IN"=w334) -> ()  [unwired: 9 in, 2 out]
            n235 = Wait (ms)(milliseconds to wait=u32 200 ("等待时间（毫秒）")) -> ()  [unwired: 1 out]
          }
          frame #4 {
            n236 = local write "工步号"(550.0 ("工步号")) -> ()
          }
        }
      }
      frame 600 {
        n237 = flat-sequence {
          tunnel: [w342] -> w336
          tunnel: w336 -> [w353]
          frame #0 {
            n238 = local read "本序合格"() -> (w347:bool)
            n239 = local read "跑合已完成次数"() -> (w340:dbl)
            n240 = Boolean To (0,1)(Boolean=w347) -> (0, 1=w351:i16)
            n241 = local read "员工姓名"() -> (w348:string)
            n242 = local read "产品ID"() -> (w341:string)
            n243 = Format Date/Time String(time format string (%c)="%Y%m%d%H%M" ("时间格式字符串(%c)")) -> (date/time string=w349:string)  [unwired: 2 in]
            n244 = Number To Decimal String(number=w351, width (-)=i16 1 ("宽度(-)")) -> (decimal integer string=w337:string)
            n245 = local read "FGCS"() -> (w344:string)
            n246 = local read "KSJJ"() -> (w346:string)
            n247 = Number To Decimal String(number=w340) -> (decimal integer string=w339:string)  [unwired: 1 in]
            n248 = Build Array(w341, w348, "1" ("元素"), w337, w346, w349, w344, "Q14070-Z050", w339) -> (w342:string[])
          }
          frame #1 {
            n249 = Wait (ms)(milliseconds to wait=u32 500 ("等待时间（毫秒）")) -> ()  [unwired: 1 out]
            n250 = call "数据库更新.vi"("设备号"="05", "数据"=w353) -> ()  [unwired: 13 in, 1 out]
          }
          frame #2 {
            n251 = local write "工步号"(660.0 ("工步号")) -> ()
          }
        }
      }
    }
    n252 = Wait Until Next ms Multiple(millisecond multiple=u32 50 ("毫秒倍数")) -> ()  [unwired: 1 out]
    n253 = local read "停止"() -> (w117:bool)
  }
  n254 = while {
    stop <- FALSE stop-if-true
    n255 = Equal?(x="密码", y="jizhuan") -> (x = y?=w359:bool)
    n256 = Compound Arithmetic op=OR(w359, "确定按钮") -> (w357:bool)
    n257 = case shown="真" w357 {
      frame False {
        w362 = T1."Disabled and Grayed Out" ("禁用")
        n258 = property on="确定按钮 3" class="Bool"("DisabledEnum"=w362) -> ()  [unwired: 2 in, 2 out]
        n259 = property on="确定按钮 2" class="Bool"("DisabledEnum"=w362) -> ()  [unwired: 2 in, 2 out]
        n260 = property on="参数修改" class="Bool (严格)"("DisabledEnum"=w362) -> ()  [unwired: 2 in, 2 out]
      }
      frame True {
        w364 = T1."Enabled" ("禁用")
        n261 = property on="确定按钮 3" class="Bool"("DisabledEnum"=w364) -> ()  [unwired: 2 in, 2 out]
        n262 = property on="确定按钮 2" class="Bool"("DisabledEnum"=w364) -> ()  [unwired: 2 in, 2 out]
        n263 = property on="参数修改" class="Bool (严格)"("DisabledEnum"=w364) -> ()  [unwired: 2 in, 2 out]
        n264 = case shown="真" "确定按钮 2" {
          frame False {
          }
          frame True {
            n265 = property on="选项卡控件 2" class="TabCtl (严格)"() -> ("Pages"=w373:refnum<vi>[])  [unwired: 2 in, 2 out]
            n266 = for {
              N: 4 -> [_]
              tunnel: w373 -> [w375] mode=indexing
              i -> [w374]
              n267 = case shown="2" w374 {
                tunnel: w375 -> [_ w377]
                frame 0, Default {
                }
                frame 2 {
                  n268 = property class="Page"(reference=w377, "PageVis"=FALSE ("选项卡可见")) -> ()  [unwired: 1 in, 2 out]
                }
              }
            }
          }
        }
        n269 = case shown="真" "确定按钮 3" {
          frame False {
          }
          frame True {
            n270 = property on="选项卡控件 2" class="TabCtl (严格)"() -> ("Pages"=w367:refnum<vi>[])  [unwired: 2 in, 2 out]
            n271 = for {
              N: 4 -> [_]
              tunnel: w367 -> [w369] mode=indexing
              i -> [w368]
              n272 = case shown="2" w368 {
                tunnel: w369 -> [_ w371]
                frame 0, Default {
                }
                frame 2 {
                  n273 = property class="Page"(reference=w371, "PageVis"=TRUE ("选项卡可见")) -> ()  [unwired: 1 in, 2 out]
                }
              }
            }
          }
        }
      }
    }
  }
  n274 = while {
    stop <- w378 stop-if-true
    n275 = stacked-sequence {
      frame #0 {
        n276 = First Call?() -> (First Call?: T/F=w380:bool)
        n277 = case shown="真" w380 {
          frame False {
          }
          frame True {
            n278 = call "员工管理测试程序.vi"() -> ("员工姓名"=w382:string, "员工ID"=w381:string)  [unwired: 10 in]
            n279 = local write "员工ID"(w381) -> ()
            n280 = local write "员工姓名"(w382) -> ()
          }
        }
      }
      frame #1 {
        n281 = local read "右极限位置(mm)"() -> (w387:dbl)
        n282 = local read "左极限位置(mm)"() -> (w386:dbl)
        n283 = local read "轴1AxisHandle OUT"() -> (w390:u32)
        n284 = local read "齿条行程(mm)"() -> (w384:dbl)
        n285 = Subtract(x=w387, y=w386) -> (x-y=w385:dbl)
        n286 = call <userlib>:"Acm_AxDiGetBit.vi"("DiChannel"=u16 3, "AxisHandle"=w390) -> ("ReturnValue"=→"ReturnValue 3":u32)  [unwired: 2 in, 3 out]
        n287 = Divide(x=w385, y=w384) -> (x/y=→"跑和百分比":dbl)
        n288 = local read "工步号"() -> (w394:dbl)
        n289 = local read "报警 工步号"() -> (w388:dbl)
        n290 = case shown="800" w394 {
          tunnel: ["联线判断" ("工步操作状态") "首先取下装钢球的辅具，准备放钢球" ("工步操作状态") "装钢球气缸顶起" ("工步操作状态") "自动放钢球启动" ("工步操作状态") "上序合格判断" ("工步操作状态") "放钢球结束" ("工步操作状态") "补钢球" ("工步操作状态") "上阻挡器放行" ("工步操作状态") "装钢球辅具放回" ("工步操作状态") "本工位在位检测" ("工步操作状态") "夹具夹紧" ("工步操作状态") "等待电机走到中间位置 " ("工步操作状态") "自制气缸夹紧" ("工步操作状态") "开始跑合" ("工步操作状态") "跑合完成" ("工步操作状态") "夹具松开" ("工步操作状态") "电机回到初始位置" ("工步操作状态") "流水线顶升气缸下降" ("工步操作状态") "本工位放行" ("工步操作状态") "放行完成" ("工步操作状态") "循环结束" ("工步操作状态") "上序不合格 ，上阻挡放行" ("工步操作状态") "本工位阻挡器放行" ("工步操作状态") "上序不合格放行完成" ("工步操作状态") "压铆力判断" ("工步操作状态") "增压缸退回" ("工步操作状态") "本序已做，请复位" ("工步操作状态") "补钢球完成" ("工步操作状态") "循环结束" ("工步操作状态")] -> w393
          frame 0, Default {
          }
          frame 5 {
          }
          frame 10 {
          }
          frame 20 {
          }
          frame 30 {
          }
          frame 40 {
          }
          frame 60 {
          }
          frame 70 {
          }
          frame 80 {
          }
          frame 90 {
          }
          frame 95 {
          }
          frame 100 {
          }
          frame 110 {
          }
          frame 120 {
          }
          frame 520 {
          }
          frame 540 {
          }
          frame 545 {
          }
          frame 550 {
          }
          frame 560 {
          }
          frame 580 {
          }
          frame 660 {
          }
          frame 700 {
          }
          frame 705 {
          }
          frame 710 {
          }
          frame 210 {
          }
          frame 211 {
          }
          frame 800 {
          }
          frame 810 {
          }
          frame 900 {
          }
        }
        "自动操作状态" <- w393
        n291 = case shown="2" w388 {
          tunnel: ["无报警" ("工步操作状态") "急停按钮被按下" ("工步操作状态") "电机报警" ("工步操作状态") "自动放钢球启动" ("工步操作状态") "放钢球" ("工步操作状态") "放钢球结束" ("工步操作状态") "补钢球" ("工步操作状态") "装钢球气缸下降" ("工步操作状态") "装钢球辅具放回" ("工步操作状态") "取拧紧辅具" ("工步操作状态") "自动拧紧启动" ("工步操作状态") "拧紧气缸下降 " ("工步操作状态") "拧紧机启动" ("工步操作状态") "拧紧气缸退回" ("工步操作状态") "拧紧辅具放回" ("工步操作状态") "测间隙启动" ("工步操作状态") "上测间隙下降" ("工步操作状态") "下测间隙上" ("工步操作状态") "下测间隙回" ("工步操作状态") "判断合格不合格" ("工步操作状态") "上测间隙回" ("工步操作状态") "压铆启动" ("工步操作状态") "增压缸快进" ("工步操作状态") "增压缸增压" ("工步操作状态") "压铆力判断" ("工步操作状态") "增压缸退回" ("工步操作状态") "不合格品，复位解除" ("工步操作状态") "补钢球完成" ("工步操作状态") "循环结束" ("工步操作状态")] -> w389
          frame 0, Default {
          }
          frame 1 {
          }
          frame 2 {
          }
          frame 20 {
          }
          frame 30 {
          }
          frame 40 {
          }
          frame 60 {
          }
          frame 70 {
          }
          frame 80 {
          }
          frame 85 {
          }
          frame 90 {
          }
          frame 100 {
          }
          frame 110 {
          }
          frame 120 {
          }
          frame 130 {
          }
          frame 140 {
          }
          frame 150 {
          }
          frame 160 {
          }
          frame 170 {
          }
          frame 175 {
          }
          frame 176 {
          }
          frame 180 {
          }
          frame 190 {
          }
          frame 200 {
          }
          frame 210 {
          }
          frame 211 {
          }
          frame 800 {
          }
          frame 810 {
          }
          frame 900 {
          }
        }
        "报警信息" <- w389
      }
      frame #2 {
        n292 = local read "拉压力（N）"() -> (w458:dbl)
        n293 = local read "电机后退"() -> (w460:bool)
        n294 = local read "电机前进"() -> (w459:bool)
        n295 = Absolute Value(x=w458) -> (abs(x)=w457:dbl)
        n296 = Not(x=w459) -> (.not. x?=w455:bool)
        n297 = Less?(x=w457, y=1000.0) -> (x < y?=w454:bool)
        n298 = Compound Arithmetic op=AND(w460, w455, w454) -> (w453:bool)
        n299 = case shown="真" w453 {
          frame False {
          }
          frame True {
            n300 = flat-sequence {
              tunnel: [w467] -> w462
              tunnel: w462 -> [w469]
              tunnel: [w469] -> w461
              tunnel: w461 -> [w470]
              tunnel: [w470] -> w463
              tunnel: w463 -> [w482]
              frame #0 {
                n301 = local read "轴1AxisHandle OUT"() -> (w464:u32)
                n302 = call "PCI1220U使能.vi"("使能"=TRUE, "AxisHandle IN"=w464) -> ()  [unwired: 9 in, 1 out]
              }
              frame #1 {
                n303 = local read "轴1AxisHandle OUT"() -> (w468:u32)
                n304 = call "PCI1220U运行.vi"("方向"=enum32{"Negative", "Positive"}."Negative" ("Direction"), "AxisHandle IN"=w468) -> ("AxisHandle OUT"=w467:u32)  [unwired: 9 in]
              }
              frame #2 {
              }
              frame #3 {
                n305 = while {
                  stop <- w474 stop-if-true
                  n306 = local read "电机后退"() -> (w481:bool)
                  n307 = local read "I急停按钮"() -> (w472:bool)
                  n308 = local read "I复位按钮"() -> (w473:bool)
                  n309 = local read "拉压力（N）"() -> (w477:dbl)
                  n310 = Not(x=w481) -> (.not. x?=w476:bool)
                  n311 = Not(x=w472) -> (.not. x?=w471:bool)
                  n312 = Wait Until Next ms Multiple(millisecond multiple=u32 50 ("毫秒倍数")) -> ()  [unwired: 1 out]
                  n313 = Absolute Value(x=w477) -> (abs(x)=w478:dbl)
                  n314 = Greater?(x=w478, y=1000.0) -> (0:w475:bool)
                  n315 = Compound Arithmetic op=OR(w476, w475, w473, w471) -> (w474:bool)
                }
              }
              frame #4 {
                n316 = call "PCI1220U停止.vi"("AxisHandle IN"=w482) -> ()  [unwired: 9 in, 2 out]
              }
            }
          }
        }
      }
      frame #3 {
        n317 = local read "拉压力（N）"() -> (w490:dbl)
        n318 = local read "电机前进"() -> (w484:bool)
        n319 = local read "电机后退"() -> (w483:bool)
        n320 = Absolute Value(x=w490) -> (abs(x)=w489:dbl)
        n321 = Not(x=w483) -> (.not. x?=w487:bool)
        n322 = Less?(x=w489, y=1000.0) -> (x < y?=w486:bool)
        n323 = Compound Arithmetic op=AND(w484, w487, w486) -> (w485:bool)
        n324 = case shown="真" w485 {
          frame False {
          }
          frame True {
            n325 = flat-sequence {
              tunnel: [w497] -> w492
              tunnel: w492 -> [w499]
              tunnel: [w499] -> w491
              tunnel: w491 -> [w500]
              tunnel: [w500] -> w493
              tunnel: w493 -> [w512]
              frame #0 {
                n326 = local read "轴1AxisHandle OUT"() -> (w495:u32)
                n327 = call "PCI1220U使能.vi"("使能"=TRUE, "AxisHandle IN"=w495) -> ()  [unwired: 9 in, 1 out]
              }
              frame #1 {
                n328 = local read "轴1AxisHandle OUT"() -> (w498:u32)
                n329 = call "PCI1220U运行.vi"("方向"=enum32{"Negative", "Positive"}."Positive" ("Direction"), "AxisHandle IN"=w498) -> ("AxisHandle OUT"=w497:u32)  [unwired: 9 in]
              }
              frame #2 {
              }
              frame #3 {
                n330 = while {
                  stop <- w505 stop-if-true
                  n331 = local read "拉压力（N）"() -> (w508:dbl)
                  n332 = local read "I急停按钮"() -> (w503:bool)
                  n333 = local read "I复位按钮"() -> (w502:bool)
                  n334 = local read "电机前进"() -> (w504:bool)
                  n335 = Not(x=w504) -> (.not. x?=w507:bool)
                  n336 = Not(x=w503) -> (.not. x?=w501:bool)
                  n337 = Absolute Value(x=w508) -> (abs(x)=w509:dbl)
                  n338 = Wait Until Next ms Multiple(millisecond multiple=u32 50 ("毫秒倍数")) -> ()  [unwired: 1 out]
                  n339 = Greater?(x=w509, y=1000.0) -> (0:w506:bool)
                  n340 = Compound Arithmetic op=OR(w507, w506, w502, w501) -> (w505:bool)
                }
              }
              frame #4 {
                n341 = call "PCI1220U停止.vi"("AxisHandle IN"=w512) -> ()  [unwired: 9 in, 2 out]
              }
            }
          }
        }
      }
    }
    n342 = Wait Until Next ms Multiple(millisecond multiple=u32 50 ("毫秒倍数")) -> ()  [unwired: 1 out]
    n343 = local read "停止"() -> (w378:bool)
  }
  n344 = flat-sequence {
    tunnel: [w514] -> w4
    tunnel: [w513] -> w3
    tunnel: w4 -> [w521]
    tunnel: w3 -> [w520]
    tunnel: [w519] -> w2
    tunnel: [w518] -> w1
    tunnel: w2 -> [w611]
    tunnel: w1 -> [w610]
    frame #0 {
      n345 = call "ADO Connection Create.vi"() -> ("error out"=w516:errorcluster, "ADODB._Connection Out"=w517:refnum<k7>)  [unwired: 10 in]
      n346 = call "ADO Connection Open.vi"("error in (no error)"=w516, "ConnectionString"="DSN=参数Z050;", "ADODB._Connection In"=w517) -> ("error out"=w513:errorcluster, "ADODB._Connection Out"=w514:refnum<k7>)  [unwired: 7 in]
      "ADODB._Connection Out" <- w514
    }
    frame #1 {
      n347 = while {
        tunnel: w521 -> [w526]
        tunnel: w520 -> [w525]
        tunnel: [w524] -> w519
        tunnel: [w523] -> w518
        stop <- w529 stop-if-true
        n348 = local read "参数加载"() -> (w522:bool)
        n349 = Wait (ms)(milliseconds to wait=u32 100 ("等待时间（毫秒）")) -> ()  [unwired: 1 out]
        n350 = First Call?() -> (First Call?: T/F=w528:bool)
        n351 = Or(x=w528, y=w522) -> (x .or. y?=w527:bool)
        n352 = case shown="真" w527 {
          tunnel: w526 -> [w532 w536]
          tunnel: w525 -> [w531 w535]
          tunnel: [w532 w534] -> w524
          tunnel: [w531 w533] -> w523
          frame False {
          }
          frame True {
            n353 = stacked-sequence {
              seq-local: [w537 _ _] -> [_ w596 _]
              tunnel: w536 -> [w539 w593 _]
              tunnel: w535 -> [w540 _ _]
              tunnel: [w539 _ _] -> w534
              tunnel: [_ w595 _] -> w533
              frame #0 {
                n354 = First Call?() -> (First Call?: T/F=w538:bool)
                n355 = case shown="真" w538 {
                  tunnel: w540 -> [w541 w546]
                  tunnel: w539 -> [_ w544]
                  tunnel: [w541 w543] -> w537
                  frame False {
                  }
                  frame True {
                    n356 = call "SQL Execute.vi"("error in (no error)"=w546, "Command Text"="SELECT * FROM 测试参数表 ;", "ADODB._Connection In"=w544) -> ("error out"=w543:errorcluster, "Data"=w547:string[][])  [unwired: 5 in, 2 out]
                    n357 = Index Array "索引数组"(array=w547, index (col)=0 ("禁用的索引 (列)")) -> (element=w550:string[])  [unwired: 1 in]
                    n358 = Array Size "数组大小"(array=w550) -> (size(s)=w549:i32)
                    n359 = while {
                      shift-right: [w555] -> w548
                      shift-left: i32[] [] -> [w556]
                      tunnel: w549 -> [w553]
                      i -> [w554]
                      stop <- w557 stop-if-true
                      n360 = Greater Or Equal?(x=w554, y=w553) -> (x >= y?=w557:bool)
                      n361 = Build Array (concatenate) "创建数组"(w556, w554) -> (w555:i32[])
                    }
                    n362 = Build Cluster Array "索引与捆绑簇数组"(w550, w548) -> (w542:cluster{"String":string, i32}[])
                    n363 = property on="型号选择" class="Ring (严格)"("StringsAndValues[]"=w542) -> ()  [unwired: 2 in, 2 out]
                  }
                }
              }
              frame #1 {
                (unwired) ",产品型号,跑合百分比,跑合次数,跑合速度,中心位置,左极限位置,右极限位置" ("查询内容")
                n364 = property on="型号选择" class="Ring (严格)"() -> ("RingText.Text"=w592:string)  [unwired: 2 in, 2 out]
                n365 = call "创建文本4"("产品型号"=w592) -> ("Result"=w594:string)  [unwired: 13 in, 1 out]
                n366 = call "SQL Execute.vi"("error in (no error)"=w596, "Command Text"=w594, "ADODB._Connection In"=w593) -> ("error out"=w595:errorcluster, "Data"=w598:string[][])  [unwired: 5 in, 2 out]
                n367 = Index Array "索引数组"(array=w598, index (row)=0 ("索引 (行)")) -> (element=w591:string[])  [unwired: 1 in]
                n368 = Fract/Exp String To Number "分数/指数字符串至数值转换"(string=w591) -> (number=w566:dbl[])  [unwired: 3 in, 1 out]
                n369 = Index Array(array=w566, index #1=1 ("索引"), index #2=2 ("索引"), index #3=3 ("索引"), index #4=4 ("索引"), index #5=5 ("索引"), index #6=6 ("索引"), index #7=7 ("索引"), index #8=8 ("索引"), index #9=9 ("索引"), index #10=10 ("索引"), index #11=11 ("索引"), index #12=12 ("索引"), index #13=13 ("索引"), index #14=14 ("索引"), index #15=15 ("索引"), index #16=16 ("索引"), index #17=17 ("索引"), index #18=18 ("索引"), index #19=19 ("索引"), index #20=20 ("索引"), index #21=21 ("索引"), index #22=22 ("索引"), index #23=23 ("索引"), index #24=24 ("索引")) -> (element #1=w565:dbl, element #2=w564:dbl, element #3=w563:dbl, element #4=w562:dbl, element #5=w561:dbl, element #6=w560:dbl, element #7=w559:dbl, element #8=w558:dbl)  [unwired: 16 out]
                n370 = local write "齿条中心位置（mm)"(w562) -> ()
                n371 = local write "左极限位置(mm)"(w561) -> ()
                n372 = local write "右极限位置(mm)"(w560) -> ()
                n373 = local write "换向拉压力(N)"(w559) -> ()
                n374 = local write "齿条行程(mm)"(w565) -> ()
                n375 = local write "跑和设定百分比"(w558) -> ()
                n376 = local write "跑合设定次数"(w564) -> ()
                n377 = local write "跑合速度(mm/s)"(w563) -> ()
              }
              frame #2 {
                n378 = local read "ADODB._Connection Out"() -> (w604:refnum<k7>)
                n379 = call "SQL Execute.vi"("Command Text"="SELECT * FROM 传感器校验表 where ID='2'", "ADODB._Connection In"=w604) -> ("Data"=w609:string[][])  [unwired: 6 in, 3 out]
                n380 = Index Array "索引数组"(array=w609) -> (element=w608:string[])  [unwired: 2 in]
                n381 = Fract/Exp String To Number "分数/指数字符串至数值转换"(string=w608) -> (number=w607:dbl[])  [unwired: 3 in, 1 out]
                n382 = Index Array "索引数组"(array=w607, index #1=1 ("索引"), index #2=2 ("索引"), index #3=3 ("索引"), index #4=4 ("索引")) -> (element #1=w600:dbl, element #2=w599:dbl)  [unwired: 2 out]
                n383 = local write "拉压力1传感器零点偏移"(w600) -> ()
                n384 = local write "拉压力1传感器比例偏移"(w599) -> ()
              }
            }
          }
        }
        n385 = local read "停止"() -> (w529:bool)
      }
    }
    frame #2 {
      n386 = call "ADO Connection Close.vi"("error in (no error)"=w610, "ADODB._Connection In"=w611) -> ("error out"=→"error out 2":errorcluster)  [unwired: 8 in, 1 out]
    }
  }
  n387 = flat-sequence {
    tunnel: [w613] -> w6
    tunnel: w6 -> [w616]
    tunnel: [w615] -> w5
    tunnel: w5 -> [w633]
    frame #0 {
      n388 = call "PCI1240U初始化.vi"() -> ("1电机"=w613:u32, "DeviceHandle"=→"DeviceHandle":u32)  [unwired: 6 in, 4 out]
      "轴1AxisHandle OUT" <- w613
    }
    frame #1 {
      n389 = while {
        tunnel: w616 -> [w629]
        tunnel: [w618] -> w615
        stop <- "停止" stop-if-true
        (unwired) "拉压力量程：5000N"
        n390 = local read "跑合速度(mm/s)"() -> (w617:dbl)
        n391 = local read "通道0"() -> (w623:dbl)
        n392 = Wait Until Next ms Multiple(millisecond multiple=u32 20 ("毫秒倍数")) -> ()  [unwired: 1 out]
        n393 = call "PCI1220电动缸速度设置.vi"("Change Velocity"=w617, "AxisHandle IN"=w629) -> ("AxisHandle OUT"=w619:u32)  [unwired: 9 in]
        n394 = local read "拉压力1传感器零点偏移"() -> (w628:dbl)
        n395 = call "PCI1220电动缸读取位置.vi"("AxisHandle IN"=w619) -> ("位置"=→"电机当前位置":dbl, "AxisHandle OUT"=w618:u32)  [unwired: 9 in]
        n396 = Divide(x=w623, y=27648.0) -> (x/y=w622:dbl)
        n397 = local read "拉压力1传感器比例偏移"() -> (w626:dbl)
        n398 = Multiply(x=w622, y=5000.0) -> (x*y=w620:dbl)
        n399 = Subtract(x=w620, y=w628) -> (x-y=w627:dbl)
        n400 = Multiply(x=w627, y=w626) -> (x*y=→"拉压力（N）":dbl)
      }
    }
    frame #2 {
      n401 = call <userlib>:"Acm_DevClose.vi"("DeviceHandle"=w633) -> ()  [unwired: 1 in, 2 out]
    }
    frame #3 {
    }
  }
